vi "Get_Randomized_Image_Name-2.vi"(2 "error IN":errorcluster, 3 "Main Name":string) -> (0 "error OUT":errorcluster, 1 "Randomized name":string)   [LabVIEW 2013]
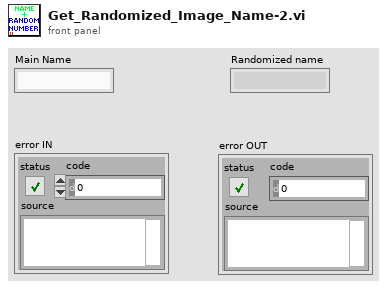
[diagram p1: front panel]
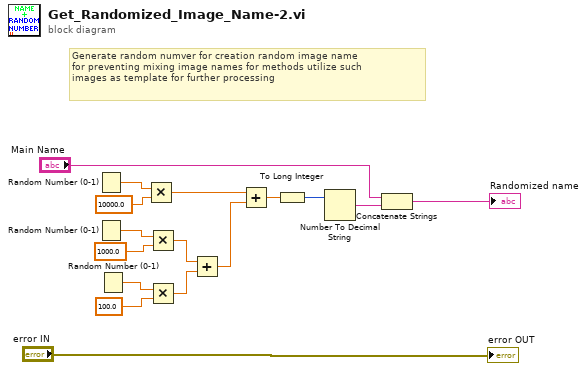
[diagram p0: block diagram]
diagram:
  # "Generate random numver for creation random image name \nfor preventing mixing image names for methods utilize such\nimages as template for further processing"
  n1 = Random Number (0-1)() -> (number: 0 to 1=w10:dbl)
  n2 = Random Number (0-1)() -> (number: 0 to 1=w9:dbl)
  n3 = Random Number (0-1)() -> (number: 0 to 1=w7:dbl)
  n4 = Multiply(x=w10, y=10000.0) -> (x*y=w3:dbl)
  n5 = Multiply(x=w9, y=1000.0) -> (x*y=w5:dbl)
  n6 = Multiply(x=w7, y=100.0) -> (x*y=w4:dbl)
  n7 = Add(x=w5, y=w4) -> (x+y=w2:dbl)
  n8 = Add(x=w3, y=w2) -> (x+y=w1:dbl)
  n9 = To Long Integer(number=w1) -> (32bit integer=w13:i32)
  n10 = Number To Decimal String(number=w13) -> (decimal integer string=w12:string)  [unwired: 1 in]
  n11 = Concatenate Strings("Main Name", w12) -> (→"Randomized name":string)
  "error OUT" <- "error IN"
